vi "Actor Core.vi"(8 "error in":errorcluster, 11 "Acquisition in":refnum<class "Acquisition.lvclass">) -> (0 "error out":errorcluster, 3 "Actor out":refnum<class "Actor.lvclass">)   [LabVIEW 2020, in "Acquisition.lvlib" / "Acquisition.lvclass"]
doc: "(<B>Filename</B>: Actor Framework.lvlib:Actor.lvclass:Actor Core.vi)\n\nReceives messages to the actor, reacts to them, and initiates any error handling that may shut the actor down.\n\nDescendant classes may override this VI to append parallel tasks for the actor to complete while it handles messages. Overrides use the Call Parent Class Method node."
uses:
  Acquisition.lvclass
  Acquisition.lvclass/Acquisition.ctl
  <vilib>/ActorFramework/Actor/Actor.lvclass
  Acquisition Messages/Acquire Msg/Acquire Msg.lvclass
  C:/Program Files (x86)/National Instruments/LabVIEW 2020/vi.lib/ActorFramework/Actor/Actor.lvclass
  D:/Storage/Source Code/Clase AF/ClaseAF/07 Aquisition AF/Acquisition/Acquisition/Acquisition.lvclass
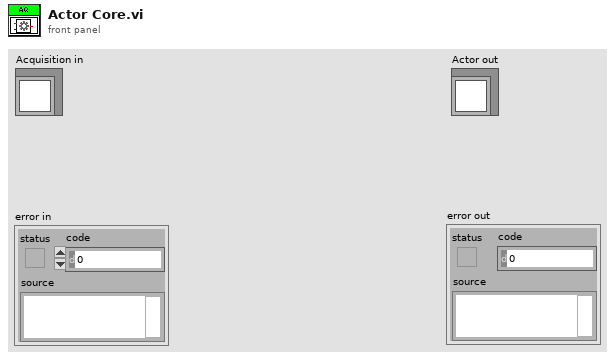
[diagram p1: front panel]
types:
  T1 = cluster{"Start":refnum<user-event>, "Stop":refnum<user-event>, "Exit":refnum<user-event>}
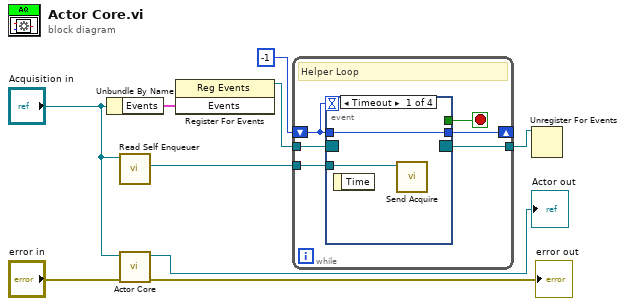
[diagram p0: block diagram]
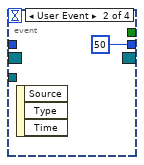
[diagram p2: hidden frame]
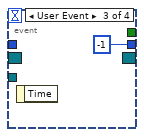
[diagram p3: hidden frame]
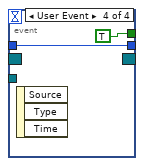
[diagram p4: hidden frame]
diagram:
  n1 = Unbundle By Name("Acquisition in") -> ("Events"=w5:T1)
  n2 = call <vilib>:"Read Self Enqueuer.vi"("Actor"="Acquisition in") -> ("Self Enqueuer"=w1:refnum<class "Message Enqueuer.lvclass">)  [unwired: 10 in]
  n3 = call-parent "Actor Core.vi"("error in"="error in", "Actor in"="Acquisition in") -> ("error out"=→"error out":errorcluster, "Actor out"=→"Actor out":refnum<class "Actor.lvclass">)  [unwired: 8 in]
  n4 = register-events(w5) -> (reference out=w6:refnum<event-registration>)  [unwired: 2 in, 1 out]
  n5 = while {
    tunnel: w6 -> [w15]
    shift-right: [w14] -> _
    shift-left: -1 -> [w11]
    tunnel: [w13] -> w3
    tunnel: w1 -> [w10]
    stop <- w12 stop-if-true
    # "Helper Loop"
    n6 = event shown="[0] Timeout" {
      selector: w15 -> [_ _ _ _]
      dyn-events: [_ _ _ _] -> w13
      timeout: w11 -> [_ _ _ _]
      tunnel: [w17 50 -1 w20] -> w14
      tunnel: [_ _ _ TRUE] -> w12
      tunnel: w11 -> [w17 _ _ w20]
      tunnel: w10 -> [w16 _ _ _]
      event Timeout {
        n7 = event-data() -> ()  [unwired: 1 in, 1 out]
        n8 = call "Send Acquire.vi"("Message Enqueuer"=w16) -> ()  [unwired: 9 in, 2 out]
      }
      event User Event {
        n9 = event-data() -> ()  [unwired: 1 in, 3 out]
      }
      event User Event {
        n10 = event-data() -> ()  [unwired: 1 in, 1 out]
      }
      event User Event {
        n11 = event-data() -> ()  [unwired: 1 in, 3 out]
      }
    }
  }
  n12 = Unregister For Events(event registration refnum=w3) -> ()  [unwired: 1 in, 1 out]
